vi "Disconnect.vi"(0 "STOMP in":refnum<class "STOMP.lvclass">, 5 "error in (no error)":errorcluster, 6 "Receipt?":bool) -> (14 "STOMP out":refnum<class "STOMP.lvclass">, 19 "error out":errorcluster)   [LabVIEW 2017, in "STOMP.lvclass"]
uses:
  STOMP.lvclass
  Typedefs/Type_ClientFrame.ctl
  Typedefs/Type_ClientFrameType.ctl
  Typedefs/Type_FrameHeader.ctl
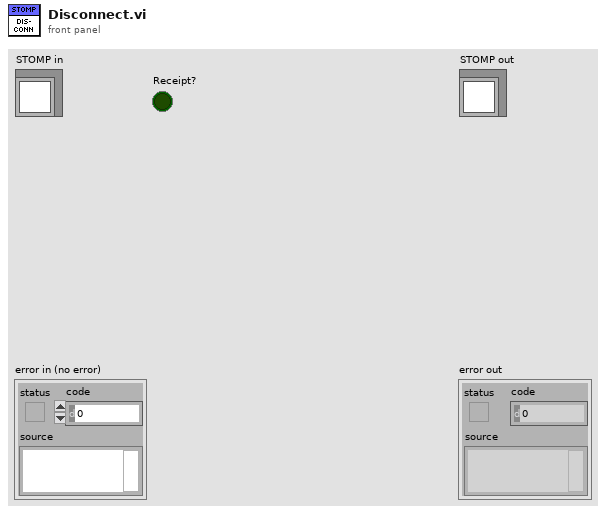
[diagram p1: front panel]
types:
  T1 = typedef "STOMP.lvclass/Type_ClientFrameType.ctl" = enum16{"Undefined", "SEND", "SUBSCRIBE", "UNSUBSCRIBE", "BEGIN", "COMMIT", "ABORT", "ACK", "NACK", "DISCONNECT"}
  T2 = typedef "STOMP.lvclass/Type_ClientFrame.ctl" = cluster{"Type":T1, "Headers":T3[], "Body":string}
  T3 = typedef "STOMP.lvclass/Type_FrameHeader.ctl" = cluster{"Header":string, "Value":string}
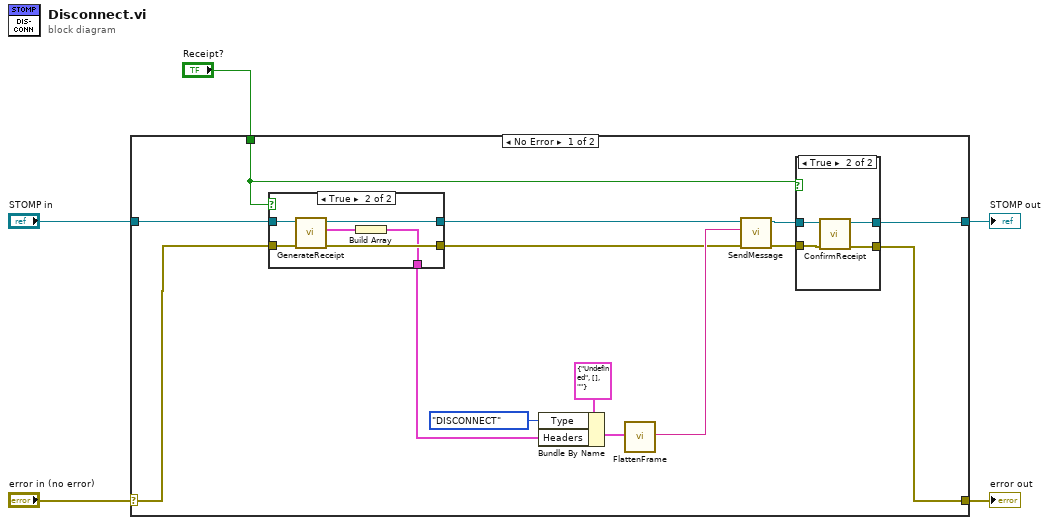
[diagram p0: block diagram]
diagram:
  n1 = case shown="No Error" "error in (no error)" {
    selector: "error in (no error)" -> [w14 w35]
    tunnel: [w9 w35] -> w4
    tunnel: [w8 w34] -> w2
    tunnel: "STOMP in" -> [w15 w34]
    tunnel: "Receipt?" -> [w7 _]
    frame No Error {
      n2 = case shown="True" w7 {
        tunnel: w15 -> [w27 w33]
        tunnel: w14 -> [w26 w32]
        tunnel: [w27 w31] -> w13
        tunnel: [w26 w30] -> w12
        tunnel: [_ w28] -> w6
        frame False {
        }
        frame True {
          n3 = call-dynamic "GenerateReceipt.vi"("error in (no error)"=w32, "STOMP in"=w33) -> ("error out"=w30:errorcluster, "Receipt Header"=w29:T3, "STOMP out"=w31:refnum<class "STOMP.lvclass">)  [unwired: 7 in]
          n4 = Build Array(w29) -> (w28:T3[])
        }
      }
      n5 = Bundle By Name(cluster=T2 {"Type"=enum."Undefined", "Headers"=[], "Body"=""} ("Type_ClientFrame"), "Type"=Type_ClientFrameType."DISCONNECT", "Headers"=w6) -> (w17:T2)
      n6 = call "FlattenFrame.vi"("Client Frame"=w17) -> ("flattened frame"=w16:string)  [unwired: 18 in]
      n7 = call-dynamic "SendMessage.vi"("error in (no error)"=w12, "data in"=w16, "STOMP in"=w13) -> ("error out"=w10:errorcluster, "STOMP out"=w11:refnum<class "STOMP.lvclass">)  [unwired: 7 in]
      n8 = case shown="True" w7 {
        tunnel: w11 -> [w20 w25]
        tunnel: w10 -> [w21 w24]
        tunnel: [w21 w23] -> w9
        tunnel: [w20 w22] -> w8
        frame False {
        }
        frame True {
          n9 = call-dynamic "ConfirmReceipt.vi"("error in (no error)"=w24, "STOMP in"=w25) -> ("error out"=w23:errorcluster, "STOMP out"=w22:refnum<class "STOMP.lvclass">)  [unwired: 8 in]
        }
      }
    }
    frame Error {
    }
  }
  "error out" <- w4
  "STOMP out" <- w2
